vi "Set google_protobuf_Enum.vi"(7 "Complete Call (T)":bool=TRUE, 8 "error in (no error)":errorcluster, 10 "package_templatemessage":T1, 11 "gRPCid":T6) -> (0 "error out":errorcluster)   [LabVIEW 2020, in "CancellableMeasurement.lvlib"]
uses:
  CancellableMeasurement.lvlib
  <vilib>/gRPC/LabVIEW gRPC Library/Shared/grpcId.ctl
  google_protobuf_Enum.ctl
  google_protobuf_EnumValue.ctl
  google_protobuf_Option.ctl
  google_protobuf_Any.ctl
  google_protobuf_SourceContext.ctl
  dcc74a39-081a-4bdd-860b-8ed792803c96.vi
  <vilib>/gRPC/LabVIEW gRPC Library/Shared/TranslateGrpcError.vi
  <vilib>/gRPC/LabVIEW gRPC Library/Server API/Server/Get Server DLL Path.vi
  <vilib>/Utility/error.llb/Error Cluster From Error Code.vi
  <vilib>/gRPC/LabVIEW gRPC Library/grpc-lvsupport-release.lvlib
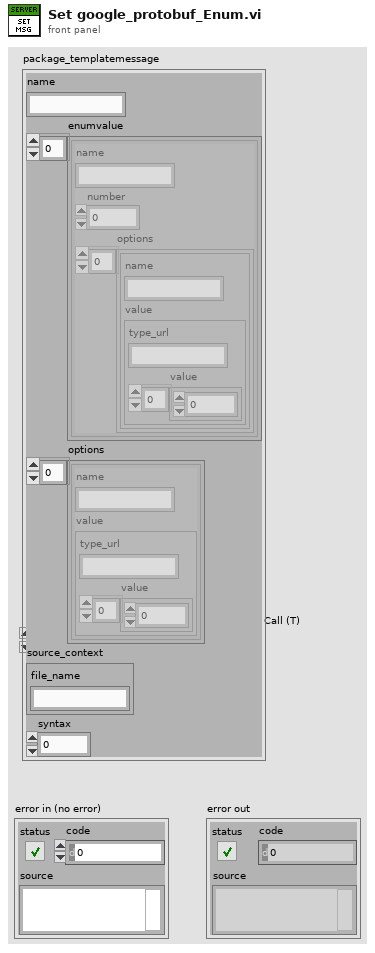
[diagram p1: front panel]
types:
  T1 = typedef "CancellableMeasurement.lvlib/google_protobuf_Enum.ctl" = cluster{"name":string, "enumvalue":T2[], "options":T3[], "source_context":T5, "syntax":i32}
  T2 = typedef "CancellableMeasurement.lvlib/google_protobuf_EnumValue.ctl" = cluster{"name":string, "number":i32, "options":T3[]}
  T3 = typedef "CancellableMeasurement.lvlib/google_protobuf_Option.ctl" = cluster{"name":string, "value":T4}
  T4 = typedef "CancellableMeasurement.lvlib/google_protobuf_Any.ctl" = cluster{"type_url":string, "value":u8[]}
  T5 = typedef "CancellableMeasurement.lvlib/google_protobuf_SourceContext.ctl" = cluster{"file_name":string}
  T6 = typedef "grpc-lvsupport-release.lvlib/grpcId.ctl" = u64
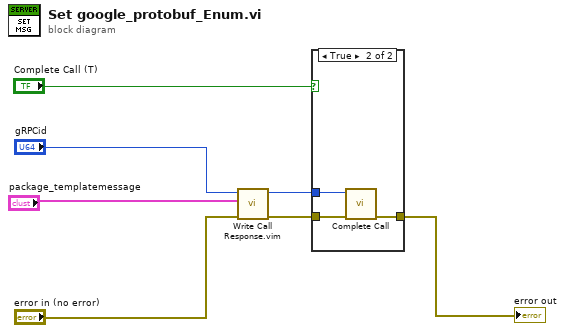
[diagram p0: block diagram]
diagram:
  n1 = call "Write Call Response.vim"("error in"="error in (no error)", "Response Data"="package_templatemessage", "gRPCid in"="gRPCid") -> ("error out"=w4:errorcluster, "gRPCid out"=w5:T6)  [unwired: 7 in]
  n2 = case shown="True" "Complete Call (T)" {
    tunnel: [w8 w11] -> w7
    tunnel: w5 -> [_ w10]
    tunnel: w4 -> [w8 w9]
    frame False {
    }
    frame True {
      n3 = call <vilib>:"Complete Call.vi"("gRPCid"=w10, "error in"=w9) -> ("error out"=w11:errorcluster)  [unwired: 8 in]
    }
  }
  "error out" <- w7
